vi "timeUnit.get.vi"(8 "error in (no error)":errorcluster, 11 "ts.relative in":refnum<class "ts.relative.lvclass">) -> (0 "error out":errorcluster, 2 "timeUnit":T1(ring), 3 "ts.relative out":refnum<class "ts.relative.lvclass">)   [LabVIEW 2020, in "ts.relative.lvclass"]
uses:
  ts.relative.lvclass
  ts.relative.lvclass/ts.relative.ctl
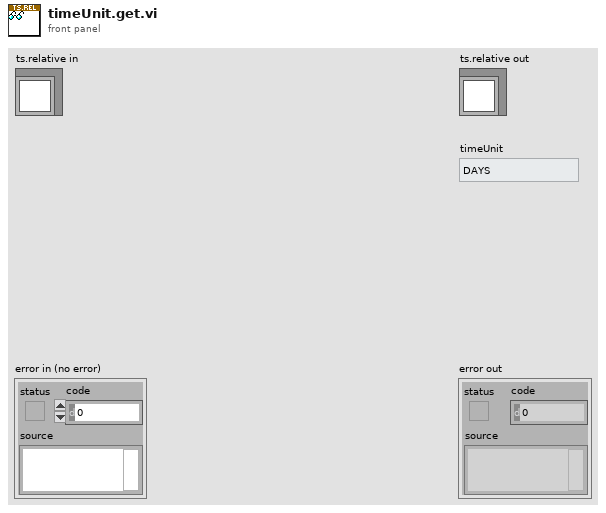
[diagram p1: front panel]
types:
  T1 = enum16{"DAYS", "HOURS", "MINUTES", "SECONDS", "MILLISECONDS", "MICROSECONDS", "NANOSECONDS", "PICOSECONDS"}
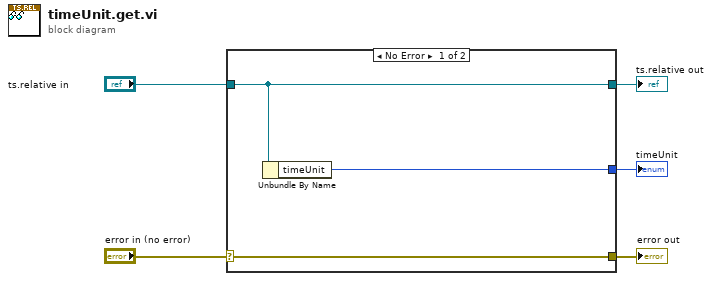
[diagram p0: block diagram]
diagram:
  n1 = case shown="No Error" "error in (no error)" {
    selector: "error in (no error)" -> [w8 w9]
    tunnel: [w8 w9] -> w4
    tunnel: [w7 w10] -> w2
    tunnel: "ts.relative in" -> [w7 w10]
    tunnel: [w6 _] -> w1
    frame No Error {
      n2 = Unbundle By Name(w7) -> ("timeUnit"=w6:T1)
    }
    frame Error {
    }
  }
  "error out" <- w4
  "ts.relative out" <- w2
  "timeUnit" <- w1
